vi "2.041 Multi-dim array-indeksering.vi"() -> ()   [LabVIEW 2022 SP3]
uses:
  <vilib>/numeric/Random Number (Range) U64.vi
  <vilib>/numeric/sub_Random U32.vi
panel:
  out "Status":string
  out "LogginSuccsess?":bool
  in  "Password":string
  in  "UserName":string
  out "transposed array":string[][](array[string])
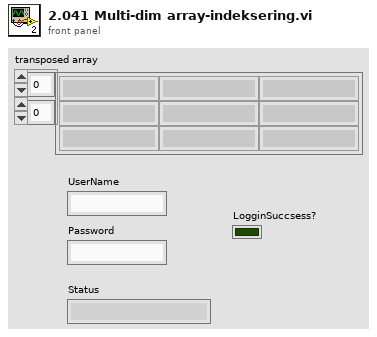
[diagram p1: front panel]
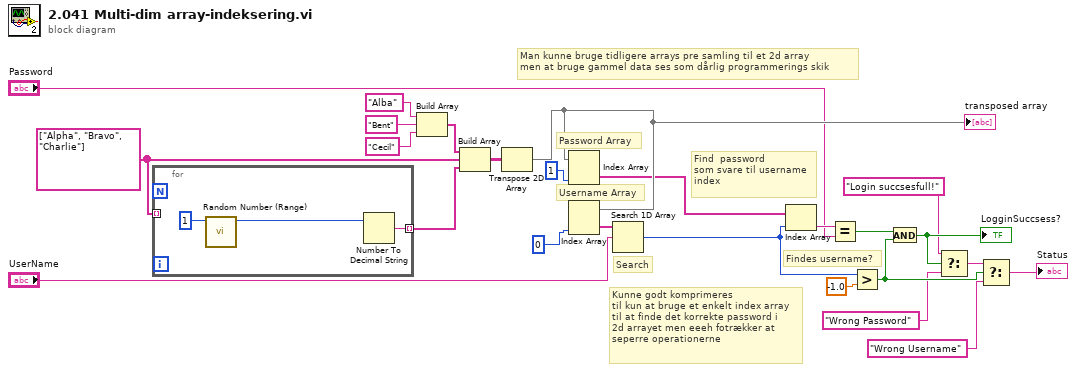
[diagram p0: block diagram]
diagram:
  w22 = string[] ["Alpha", "Bravo", "Charlie"]
  # "Kunne godt komprimeres\ntil kun at bruge et enkelt index array\ntil at finde det korrekte password i \n2d arrayet men eeeh fotrækker at\nseperre operationerne"
  # "Man kunne bruge tidligere arrays pre samling til et 2d array \nmen at bruge gammel data ses som dårlig programmerings skik"
  # "Find  password\nsom svare til username\nindex"
  # "Findes username?"
  # "Search"
  # "Username Array"
  # "Password Array"
  n1 = for {
    tunnel: w22 -> [_] mode=indexing
    tunnel: [w26] -> w21 mode=indexing
    n2 = call-poly <vilib>:"Random Number (Range).vi"("upper bound (100)"=u64 1) -> ("number"=w27:u64)  [unwired: 10 in]
    n3 = Number To Decimal String(number=w27) -> (decimal integer string=w26:string)  [unwired: 1 in]
  }
  n4 = Build Array("Alba", "Bent", "Cecil") -> (w19:string[])
  n5 = Build Array(w19, w22, w21) -> (w20:string[][])
  n6 = Transpose 2D Array(2D array=w20) -> (transposed array=w15:string[][])
  "transposed array" <- w15
  n7 = Index Array(array=w15, index (col)=1 ("index (row)")) -> (element=w14:string[])  [unwired: 1 in]
  n8 = Index Array(array=w15, index (col)=0 ("index (row)")) -> (element=w18:string[])  [unwired: 1 in]
  n9 = Search 1D Array(1D array=w18, element="UserName") -> (index of element=w10:i32)  [unwired: 1 in]
  n10 = Index Array(array=w14, index=w10) -> (element=w13:string)
  n11 = Equal?(x=w13, y="Password") -> (x = y?=w9:bool)
  n12 = Greater?(x=w10, y=-1.0) -> (0:w8:bool)
  n13 = And(x=w9, y=w8) -> (x .and. y?=w7:bool)
  "LogginSuccsess?" <- w7
  n14 = Select(t="Login succsesfull!", s=w7, f="Wrong Password") -> (s? t:f=w4:string)
  n15 = Select(t=w4, s=w8, f="Wrong Username") -> (s? t:f=→"Status":string)
